vi "Untitled 1.vi"() -> ()   [LabVIEW 2020]
panel:
  out "s? t:f":dbl[](array[numeric])
  in  "Boolean":bool
  in  "Interaçôes":i32
  out "Slide":dbl(slide) scale=0.0..100.0
  in  "Array 2 - 0":dbl
  in  "Numeric 3":dbl
  out "i- Value":i32
  in  "Array 1 - 1":dbl
  in  "Array 1 - 0":dbl
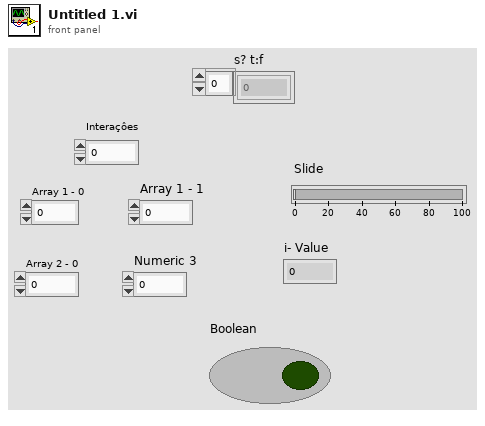
[diagram p1: front panel]
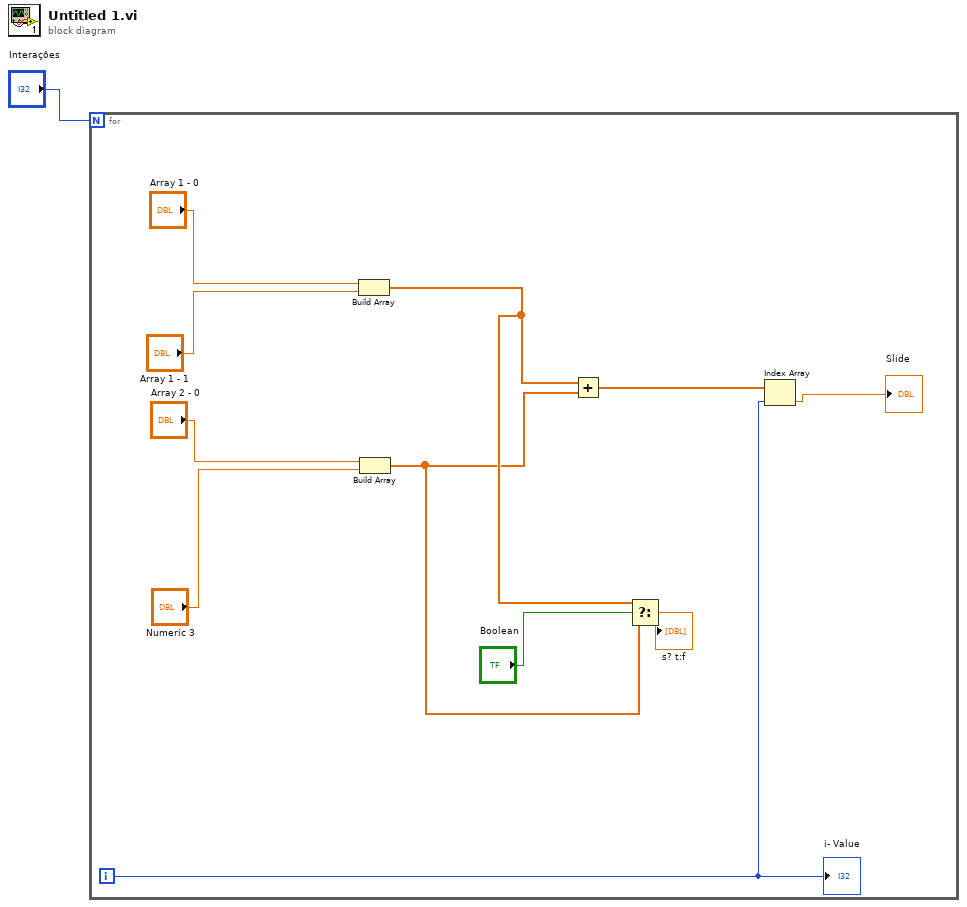
[diagram p0: block diagram]
diagram:
  n1 = for {
    N: "Interaçôes" -> [_]
    i -> [w6]
    n2 = Build Array("Array 1 - 0", "Array 1 - 1") -> (w5:dbl[])
    n3 = Build Array("Array 2 - 0", "Numeric 3") -> (w4:dbl[])
    n4 = Add(x=w5, y=w4) -> (x+y=w8:dbl[])
    n5 = Select(t=w5, s="Boolean", f=w4) -> (s? t:f=→"s? t:f":dbl[])
    n6 = Index Array(array=w8, index=w6) -> (element=→"Slide":dbl)
    "i- Value" <- w6
  }
